vi "Write Target State.vi"(10 "Target State":refnum<class "state.lvclass">, 11 "statemachine in":refnum<class "statemachine.lvclass">) -> (3 "statemachine out":refnum<class "statemachine.lvclass">)   [LabVIEW 2020, in "eos.lvlib" / "statemachine.lvclass"]
uses:
  statemachine.lvclass
  interfaces/state/state.lvclass
  statemachine.lvclass/statemachine.ctl
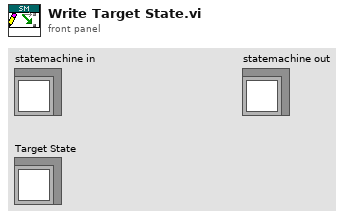
[diagram p1: front panel]
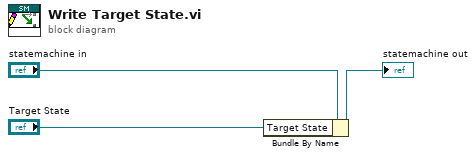
[diagram p0: block diagram]
diagram:
  n1 = Bundle By Name(cluster="statemachine in", "Target State"="Target State") -> (→"statemachine out":refnum<class "statemachine.lvclass">)
